vi "midi-track.get_with_timing.vi"(8 "error in (no error)":errorcluster, 10 "Track Number":i32, 11 "midi-file-events in":refnum<class "midi-file-events.lvclass">) -> (0 "error out":errorcluster, 2 "Events by time":T1(c390), 3 "midi-file-events out":refnum<class "midi-file-events.lvclass">)   [LabVIEW 2020, in "midi-file-events.lvclass"]
uses:
  midi-file-events.lvclass
  midi-file-event.midi/midi-file-event.midi.lvclass
  midi-file-events.lvclass/midi-file-events.ctl
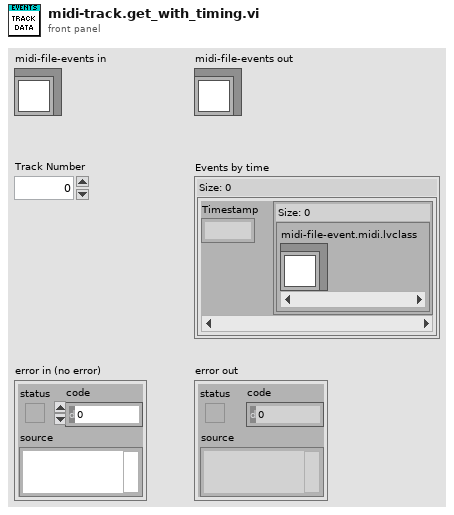
[diagram p1: front panel]
types:
  T1 = map{dbl, set{refnum<class "midi-file-event.midi.lvclass">}}
  T2 = typedef "midi-file-events.lvclass/privatedata.ctl" = cluster{"ticks per quarter note (division)":i16, "Tempo Map":map{dbl, dbl}, "Track data by Track number":map{i32, map{dbl, set{refnum<class "midi-file-event.midi.lvclass">}}}}
  T3 = map{i32, map{dbl, set{refnum<class "midi-file-event.midi.lvclass">}}}
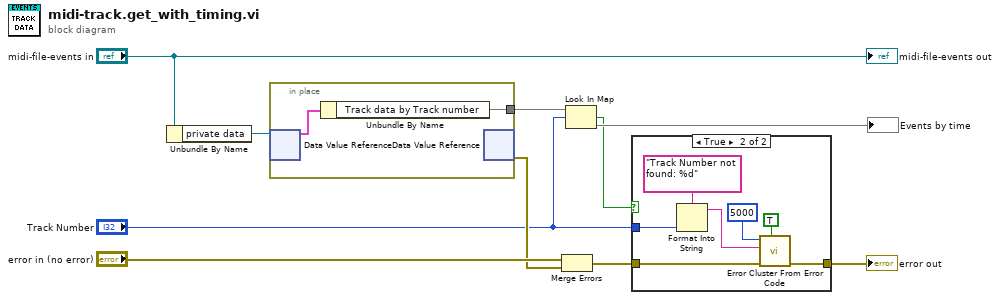
[diagram p0: block diagram]
diagram:
  n1 = Unbundle By Name("midi-file-events in") -> ("private data"=w10:refnum<data-value>)
  n2 = in-place {
    in-place-border: [w11] -> w9
    n3 = in-place-dvr #1(w10) -> (w12:T2)  [unwired: 1 out]
    n4 = Unbundle By Name(w12) -> ("Track data by Track number"=w11:T3)
    n5 = in-place-dvr #1() -> (w6:errorcluster)  [unwired: 1 in, 1 out]
  }
  n6 = Merge Errors("error in (no error)", w6) -> (w4:errorcluster)
  n7 = Look In Map(map=w9, key="Track Number") -> (key not found?=w1:bool, value=→"Events by time":T1)  [unwired: 1 in]
  n8 = case shown="True" w1 {
    tunnel: "Track Number" -> [_ w19]
    tunnel: w4 -> [w13 w15]
    tunnel: [w13 w14] -> w3
    frame False {
    }
    frame True {
      n9 = Format Into String(format string="Track Number not found: %d", w19) -> (resulting string=w16:string)  [unwired: 2 in, 1 out]
      n10 = call <vilib>:"Error Cluster From Error Code.vi"("show call chain? (False)"=TRUE, "error in (no error)"=w15, "error message (\"\")"=w16, "error code (0)"=5000) -> ("error out"=w14:errorcluster)  [unwired: 5 in]
    }
  }
  "error out" <- w3
  "midi-file-events out" <- "midi-file-events in"
